vi "MT Rayleigh Fading Profile (Gans).vi"(0 "profile length (samples)":i32=1000, 5 "sampling frequency (Hz)":dbl=1.0 format="%.2f", 7 "doppler spread (Hz)":dbl=0.01 format="%.2p", 9 "seed in (0xFFFFFFFF)":i32=-1 format="%.0x", 11 "error in (no error)":errorcluster, 12 "fading variance":dbl=1.0 format="%.2f", 13 "reset? (T)":bool=TRUE) -> (4 "fading profile":cdb[](array[numeric]) format="%.2f", 10 "seed out":i32 format="%.0x", 15 "error out":errorcluster)   [LabVIEW 2020, in "niDMT.lvlib"]
doc: "This polymorphic instance generates a Rayleigh flat-fading profile with an envelope that statistically obeys the Rayleigh distribution, using the Gans fading model."
uses:
  <vilib>/addons/Modulation/niDMT.lvlib
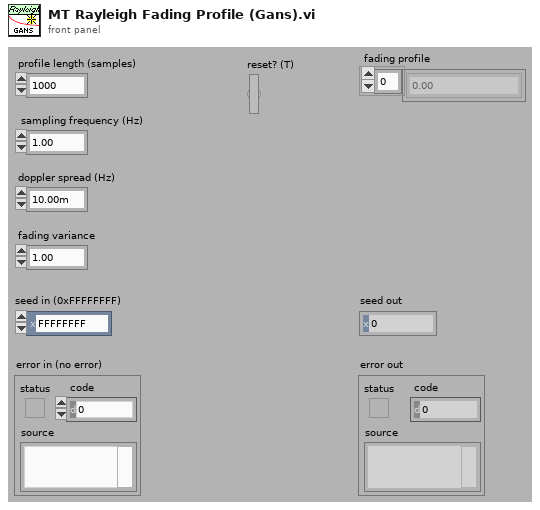
[diagram p1: front panel]
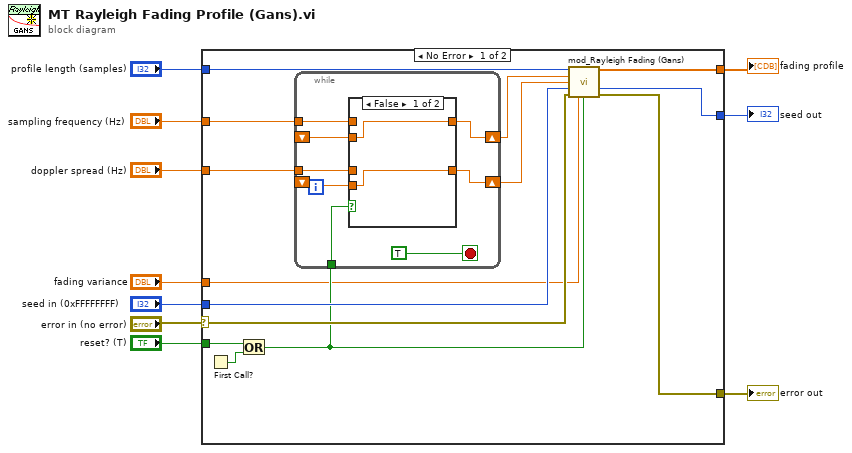
[diagram p0: block diagram]
diagram:
  n1 = case shown="No Error" "error in (no error)" {
    selector: "error in (no error)" -> [w21 w37]
    tunnel: "profile length (samples)" -> [w22 _]
    tunnel: [w24 _] -> w9
    tunnel: [w23 w37] -> w8
    tunnel: "sampling frequency (Hz)" -> [w16 _]
    tunnel: "doppler spread (Hz)" -> [w15 _]
    tunnel: "fading variance" -> [w12 _]
    tunnel: "reset? (T)" -> [w20 _]
    tunnel: "seed in (0xFFFFFFFF)" -> [w18 _]
    tunnel: [w11 _] -> w1
    frame No Error {
      n2 = First Call?() -> (First Call?: T/F=w19:bool)
      n3 = Or(x=w20, y=w19) -> (x .or. y?=w17:bool)
      n4 = while {
        tunnel: w17 -> [w31]
        tunnel: w16 -> [w30]
        shift-right: [w29] -> w14
        shift-left: _ -> [w28]
        tunnel: w15 -> [w27]
        shift-right: [w26] -> w13
        shift-left: _ -> [w25]
        stop <- TRUE stop-if-true
        n5 = case shown="False" w31 {
          tunnel: w30 -> [_ w36]
          tunnel: [w34 w36] -> w29
          tunnel: w28 -> [w34 _]
          tunnel: w27 -> [_ w35]
          tunnel: [w33 w35] -> w26
          tunnel: w25 -> [w33 _]
          frame False {
          }
          frame True {
          }
        }
      }
      n6 = call <vilib>:"mod_Rayleigh Fading (Gans).vi"("profile length (samples)"=w22, "sampling frequency (Hz)"=w14, "doppler spread (Hz)"=w13, "seed in (0xFFFFFFFF)"=w18, "error in (no error)"=w21, "fading variance"=w12, "reset? (T)"=w17) -> ("rayleigh fading profile"=w24:cdb[], "seed out"=w11:i32, "error out"=w23:errorcluster)  [unwired: 6 out]
    }
    frame Error {
    }
  }
  "fading profile" <- w9
  "error out" <- w8
  "seed out" <- w1
